vi "Create User Events.vi"(8 "Error In":errorcluster) -> (0 "Error Out":errorcluster, 3 "Event Registration Refnum":refnum<event-registration>)   [LabVIEW 2020]
doc: "Create a boolean user event that will be used to stop the event loop from the message handling loop."
uses:
  Typedefs/Top level VI states.ctl
  Global Variables/gl_User Events.vi
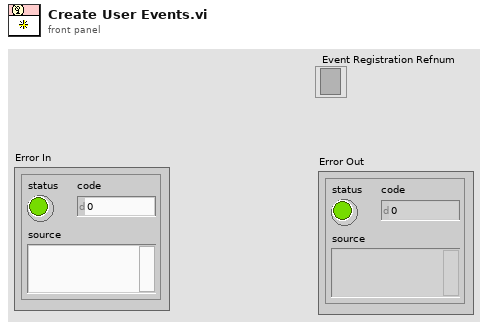
[diagram p1: front panel]
types:
  T1 = typedef "Top level VI states.ctl" = enum16{"None", "Initialise UI", "<STACK PROTOCOL STATES>", "AOL Zstack-START", "AOL Zstack-STOP", "Motor Zstack-START", "Motor Zstack-STOP", "<ACQUISITION PROTOCOL STATES> ", "Functional Acquisition-START", "Functional Acquisition-STOP", "Single Plane Acquisition-START", "Single Plane Acquisition-STOP", "Volume Acquisition-START", "Volume Acquisition-STOP", "<LIVE IMAGING PROTOCOL STATES>", "Live Imaging-START", "Live Imaging-STOP", "Live Plane Imaging-START", "Live Plane Imaging-STOP", "Live Volume Imaging-START", "Live Volume Imaging-STOP", "<MOVEMENT CORRECTION PROTOCOL STATES>", "EXIT"}
  T2 = cluster{"Stop":refnum<user-event>, "Next State":refnum<user-event>}
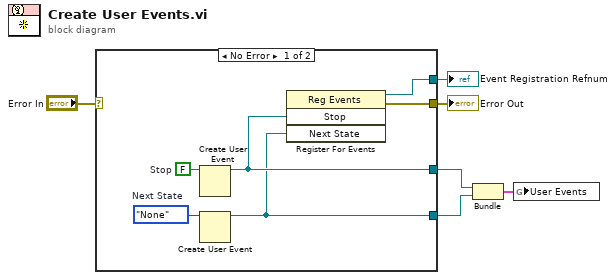
[diagram p0: block diagram]
diagram:
  n1 = case shown="No Error" "Error In" {
    selector: "Error In" -> [_ w13]
    tunnel: [w12 _] -> w4
    tunnel: [w11 _] -> w1
    tunnel: [w10 w13] -> w5
    tunnel: [w8 _] -> w3
    frame No Error {
      w7 = Top_level_VI_states."None"  # Next State
      w9 = FALSE  # Stop
      n2 = Create User Event(user event datatype=w9) -> (user event=w12:refnum<user-event>)  [unwired: 1 in, 1 out]
      n3 = Create User Event(user event datatype=w7) -> (user event=w8:refnum<user-event>)  [unwired: 1 in, 1 out]
      n4 = register-events(w12, w8) -> (reference out=w11:refnum<event-registration>, error out=w10:errorcluster)  [unwired: 2 in]
    }
    frame Error {
    }
  }
  "Error Out" <- w5
  "Event Registration Refnum" <- w1
  n5 = Bundle("Stop"=w4, "Next State"=w3) -> (w2:T2)  [unwired: 1 in]
  n6 = global write "gl_User Events.vi" "User Events"(w2) -> ()
